vi "Questão 1.vi"() -> ()   [LabVIEW 2019]
uses:
  <vilib>/measure/matone.llb/Extract Multiple Tone Information 1 Chan.vi
  <vilib>/measure/NI_MAPro.lvlib
panel:
  in  "file path 2":path=path "C:/lista3.tdms"
  in  "file path":path=path "C:/lista2.tdms"
  out "Waveform Graph 8":dynamicdata(graph)
  out "Waveform Graph 7":dynamicdata(graph)
  out "Waveform Graph 6":dynamicdata(graph)
  out "Waveform Graph 2":dynamicdata(graph)
  out "multiple tone information":T1(array[cluster]) {"detected phase (deg)" format="%_6g"; "detected amplitude" format="%_6p"; "detected frequency" format="%_6p"}
  out "Waveform Graph 4":waveform(dbl)(graph)
  out "Waveform Graph 3":waveform(dbl)(graph)
  in  "Phase 3":dbl caption="Phase"
  in  "Amplitude 3":dbl=0.5 caption="Amplitude"
  in  "Frequency 3":dbl=40.0 caption="Frequency"
  in  "Phase 2":dbl caption="Phase"
  in  "Amplitude 2":dbl=1.0 caption="Amplitude"
  in  "Frequency 2":dbl=20.0 caption="Frequency"
  in  "Phase":dbl
  in  "Amplitude":dbl=2.0
  in  "Frequency":dbl=10.0
  out "Waveform Graph":dynamicdata(graph)
  # "Phase em graus"
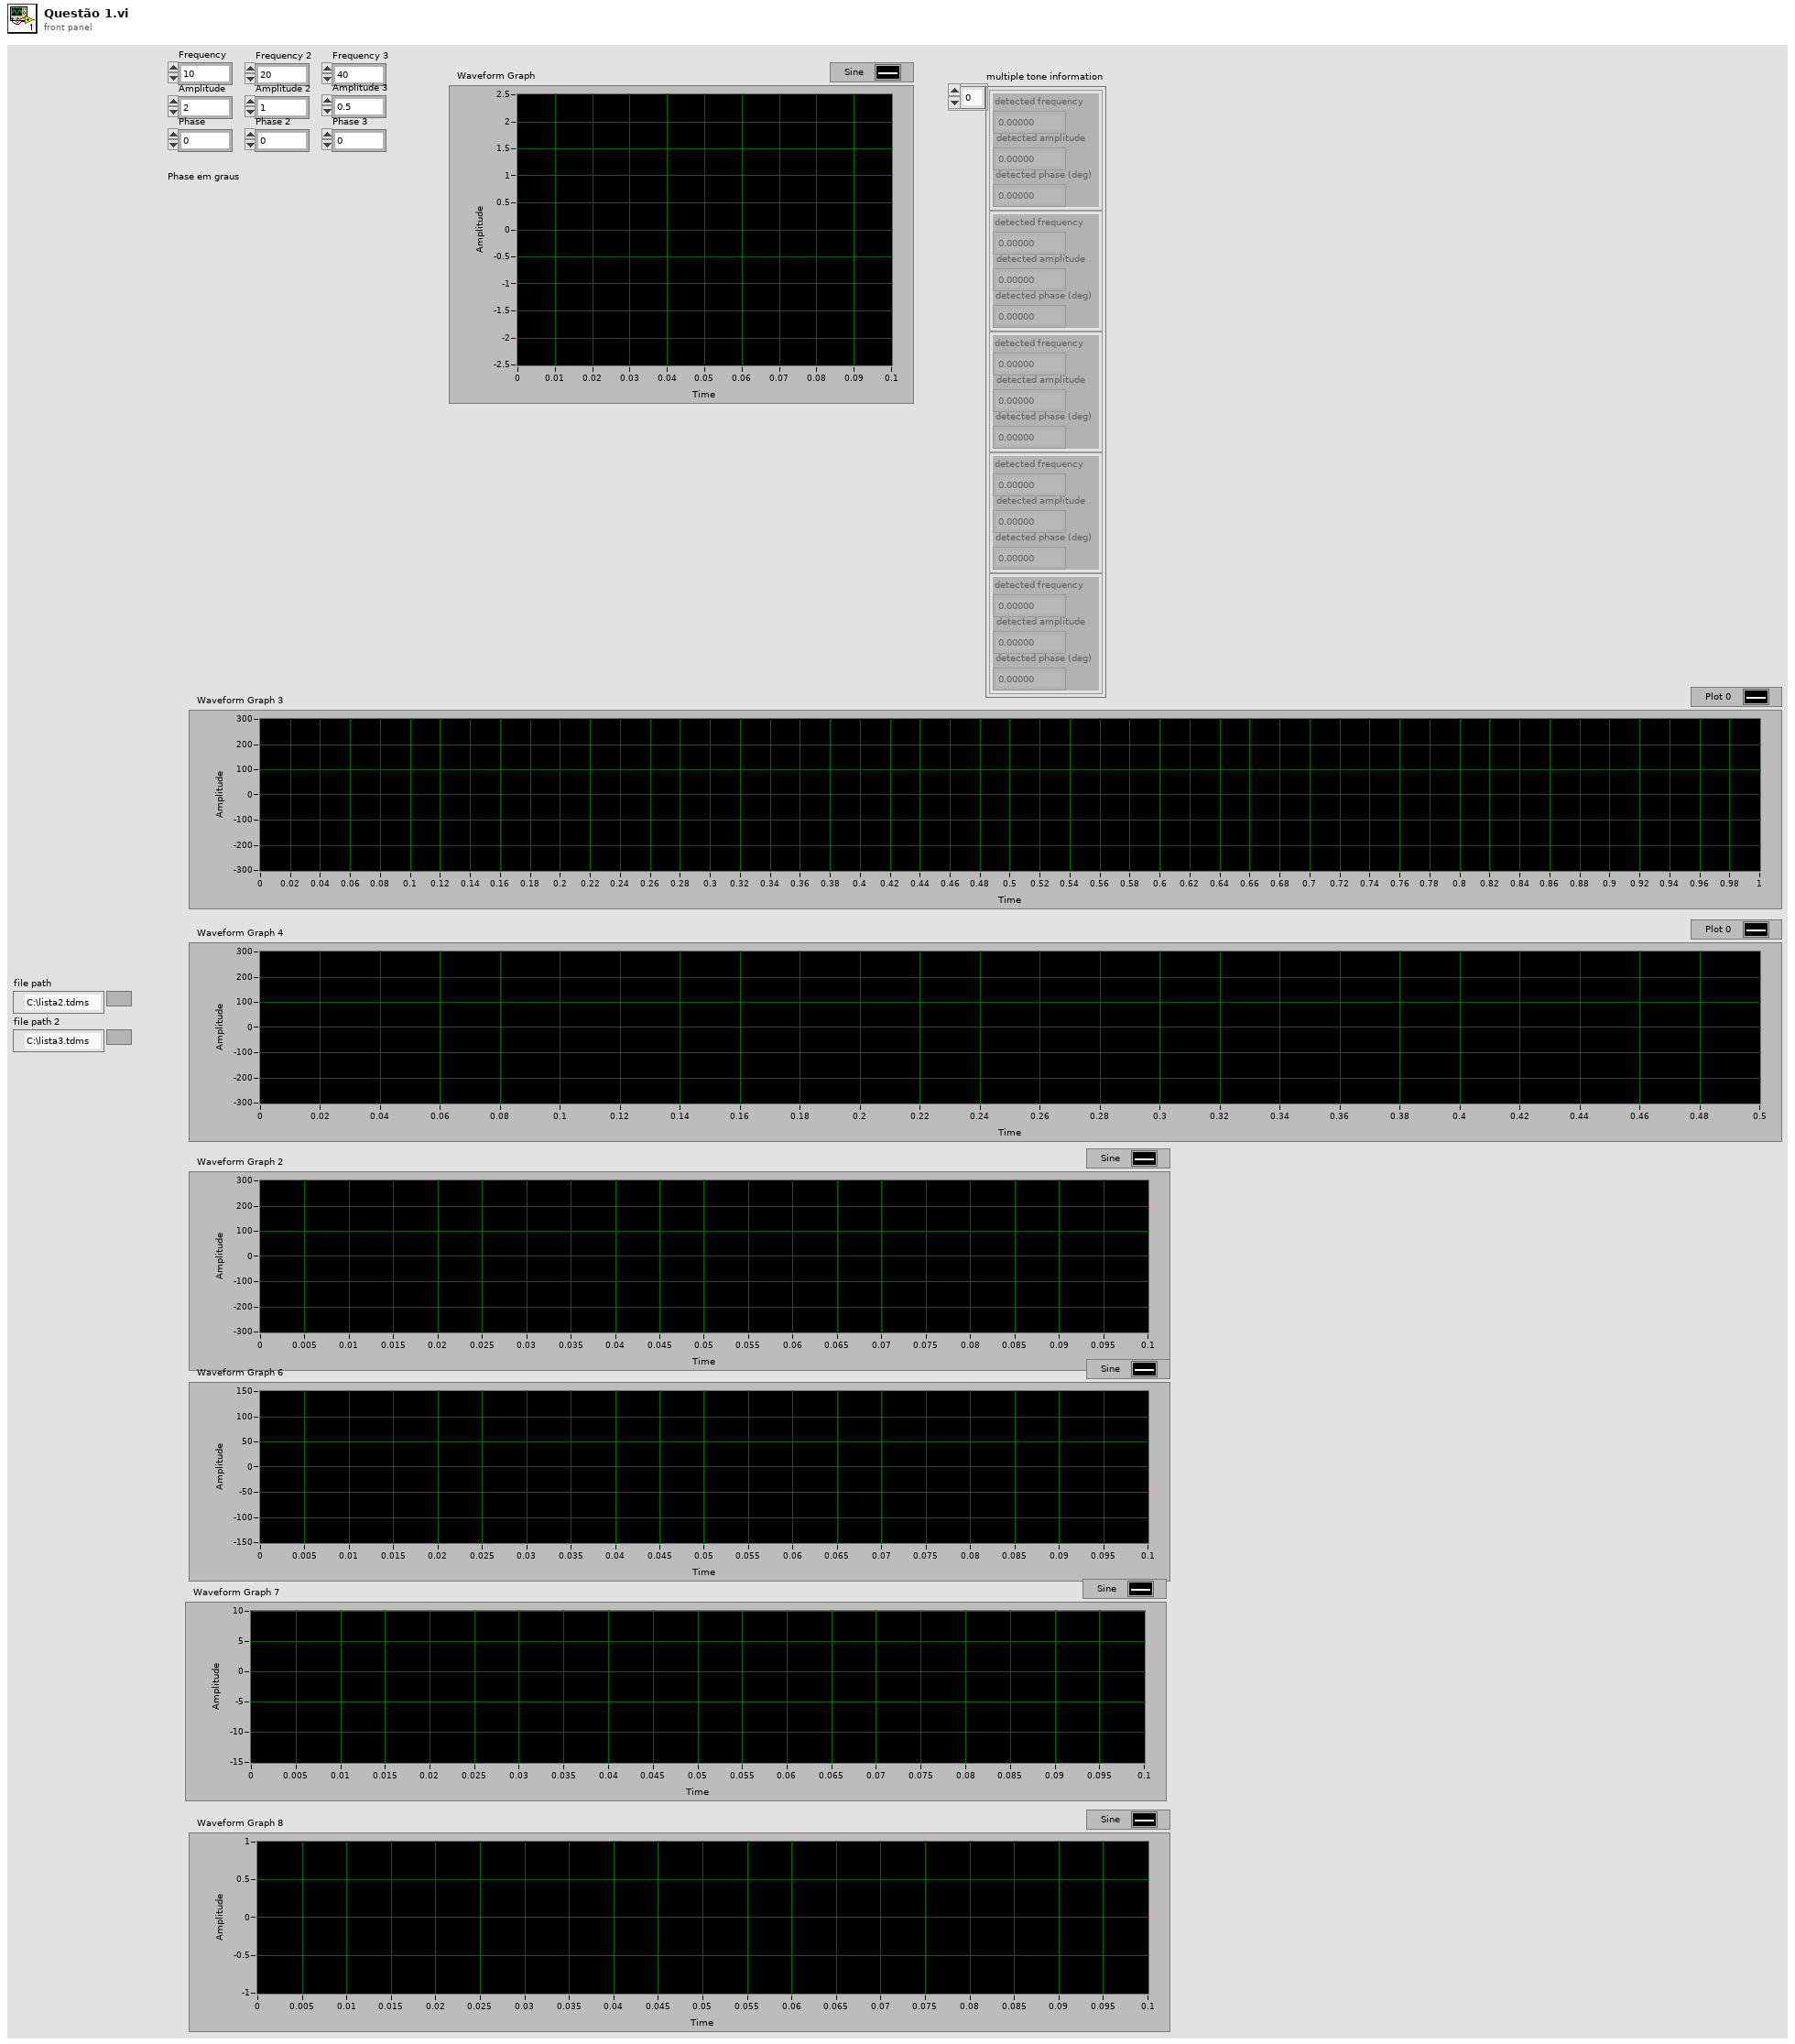
[diagram p1: front panel]
types:
  T1 = cluster{"detected frequency":dbl, "detected amplitude":dbl, "detected phase (deg)":dbl}[]
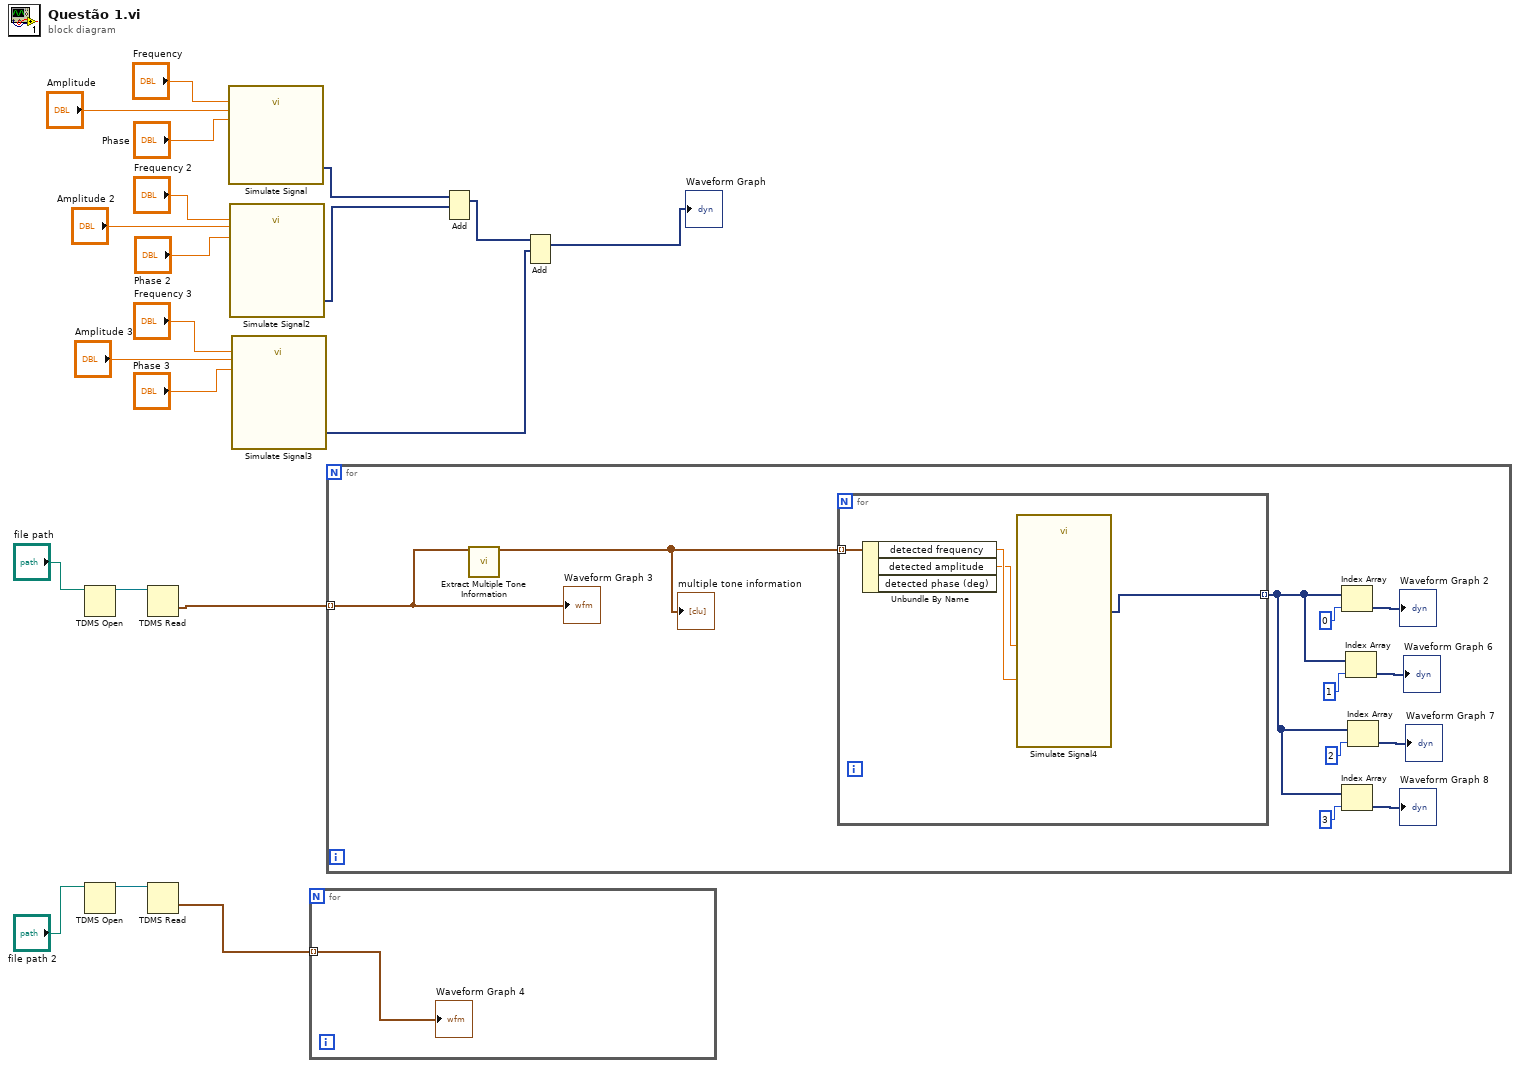
[diagram p0: block diagram]
diagram:
  n1 = TDMS Open(11:"file path") -> (3:w19:refnum<k34>)  [unwired: 6 in, 1 out]
  n2 = TDMS Open(11:"file path 2") -> (3:w17:refnum<k34>)  [unwired: 6 in, 1 out]
  n3 = TDMS Read(0:w19) -> (10:w15:waveform(dbl)[])  [unwired: 7 in, 5 out]
  n4 = TDMS Read(0:w17) -> (10:w16:waveform(dbl)[])  [unwired: 7 in, 5 out]
  n5 = call "Simulate Signal"("Frequency"="Frequency", "Amplitude"="Amplitude", "Phase"="Phase") -> ("Sine"=w1:dynamicdata)  [unwired: 11 in, 1 out]
  n6 = call "Simulate Signal2"("Frequency"="Frequency 2", "Amplitude"="Amplitude 2", "Phase"="Phase 2") -> ("Sine"=w2:dynamicdata)  [unwired: 11 in, 1 out]
  n7 = call "Simulate Signal3"("Frequency"="Frequency 3", "Amplitude"="Amplitude 3", "Phase"="Phase 3") -> ("Sine"=w4:dynamicdata)  [unwired: 11 in, 1 out]
  n8 = for {
    tunnel: w16 -> [w21] mode=indexing
    "Waveform Graph 4" <- w21
  }
  n9 = for {
    tunnel: w15 -> [w32] mode=indexing
    n10 = call-poly <vilib>:"Extract Multiple Tone Information.vi"("time signal in"=w32) -> ("multiple tone information"=w31:T1)  [unwired: 12 in, 2 out]
    "multiple tone information" <- w31
    n11 = for {
      tunnel: w31 -> [w36] mode=indexing
      tunnel: [w33] -> w22 mode=indexing
      n12 = Unbundle By Name(w36) -> ("detected frequency"=w35:dbl, "detected amplitude"=w34:dbl)  [unwired: 1 out]
      n13 = call "Simulate Signal4"("Frequency"=w35, "Amplitude"=w34) -> ("Sine"=w33:dynamicdata)  [unwired: 12 in, 1 out]
    }
    n14 = Index Array(array=w22, index=0) -> (element=→"Waveform Graph 2":dynamicdata)
    n15 = Index Array(array=w22, index=3) -> (element=→"Waveform Graph 8":dynamicdata)
    n16 = Index Array(array=w22, index=1) -> (element=→"Waveform Graph 6":dynamicdata)
    n17 = Index Array(array=w22, index=2) -> (element=→"Waveform Graph 7":dynamicdata)
    "Waveform Graph 3" <- w32
  }
  n18 = Add(1:w2, 2:w1) -> (0:w3:dynamicdata)  [unwired: 1 in, 1 out]
  n19 = Add(1:w4, 2:w3) -> (0:→"Waveform Graph":dynamicdata)  [unwired: 1 in, 1 out]
